vi "离线通道切换频率.vi"(8 "错误输入":errorcluster caption="输出簇", 11 "文件句柄":i32) -> (0 "错误输出":errorcluster, 2 "采集频率":dbl, 3 "文件句柄出":i32)   [LabVIEW 2011]
uses:
  dll/em9636.dll
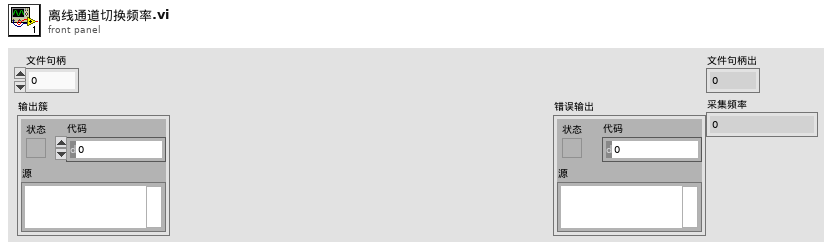
[diagram p1: front panel]
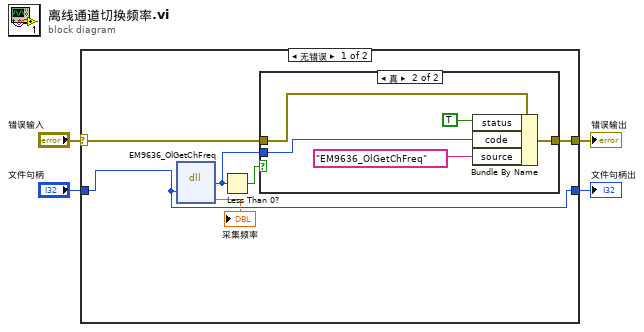
[diagram p0: block diagram]
diagram:
  n1 = case shown="无错误" "错误输入" {
    selector: "错误输入" -> [w6 w18]
    tunnel: [w8 w18] -> w3
    tunnel: "文件句柄" -> [w7 w17]
    tunnel: [w7 w17] -> w1
    frame No Error {
      n2 = dll-call lib="PTH1abs Eèµ éç LABVIEWæºVI(v2.0)EM9636BD)EM9636BDè°ç¨APIå½æ°æ¹æ³éè®¯ä¾ç¨EM9636_demo_labview2011dll\nem9636.dll" fn="EM9636_OlGetChFreq"("文件句柄"=w7) -> ("错误信息"=w9:i32, "通道切换频率值"=→"采集频率":dbl)  [unwired: 5 in, 2 out]
      n3 = Less Than 0?(x=w9) -> (x < 0?=w10:bool)
      n4 = case shown="真" w10 {
        tunnel: [w11 w14] -> w8
        tunnel: w6 -> [w11 w16]
        tunnel: w9 -> [_ w13]
        frame False {
        }
        frame True {
          n5 = Bundle By Name(cluster=w16, "status"=TRUE, "code"=w13, "source"="EM9636_OlGetChFreq") -> (w14:errorcluster)
        }
      }
    }
    frame Error {
    }
  }
  "文件句柄出" <- w1
  "错误输出" <- w3
